vi "Query Power Analysis Setting.vi"(8 "error in (no error)":errorcluster, 10 "Setting Type (0: Control Loop Response)":i32(ring) items=["Control Loop Response", "Power Supply Rejection Ratio"], 11 "VISA resource name":refnum<visa-resource-name>) -> (0 "error out":errorcluster, 2 "Setting Information":string, 3 "VISA resource name out":refnum<visa-resource-name>)   [LabVIEW 2015, in "Agilent 2000 3000 X-Series.lvlib"]
doc: "Returns the power analysis settings. \n\n<b>Note:</b>\nThis VI is only applicable for 3000T, 4000, 6000 X-Series."
uses:
  Agilent 2000 3000 X-Series.lvlib
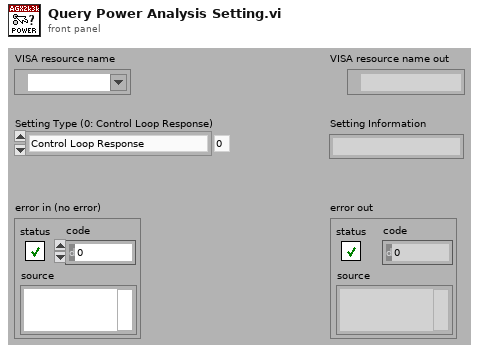
[diagram p1: front panel]
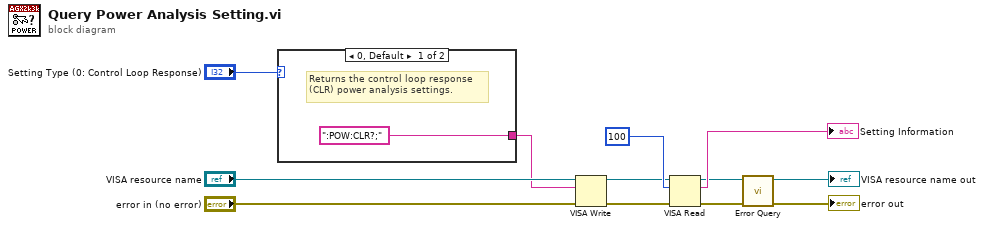
[diagram p0: block diagram]
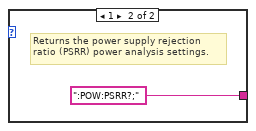
[diagram p2: hidden frame]
diagram:
  n1 = case shown="0, Default" "Setting Type (0: Control Loop Response)" {
    tunnel: [":POW:CLR?;" ":POW:PSRR?;"] -> w5
    frame 0, Default {
      # "Returns the control loop response\n(CLR) power analysis settings."
    }
    frame 1 {
      # "Returns the power supply rejection \nratio (PSRR) power analysis settings."
    }
  }
  n2 = VISA Write(VISA resource name="VISA resource name", write buffer=w5, error in (no error)="error in (no error)") -> (VISA resource name out=w9:refnum<visa-resource-name>, error out=w8:errorcluster)  [unwired: 1 out]
  n3 = VISA Read(VISA resource name=w9, byte count=100, error in (no error)=w8) -> (VISA resource name out=w3:refnum<visa-resource-name>, read buffer=→"Setting Information":string, error out=w4:errorcluster)  [unwired: 1 out]
  n4 = call "Error Query.vi"("error in (no error)"=w4, "VISA resource name"=w3) -> ("error out"=→"error out":errorcluster, "VISA resource name out"=→"VISA resource name out":refnum<visa-resource-name>)  [unwired: 6 in, 2 out]
